vi "Get Output Uncertainty.vi"(8 "error in (no error)":errorcluster, 9 "Specified Uncertainty (0: 90-days)":u32(ring) items=["90-days", "365-days"], 10 "Output (T: Primary)":bool=TRUE, 11 "VISA resource name":refnum<visa-resource-name>) -> (0 "error out":errorcluster, 1 "Output Uncertainty Units":i32, 2 "Output Uncertainty":dbl format="%.4f", 3 "VISA resource name out":refnum<visa-resource-name>, 4 "Specification Interval":i32)   [LabVIEW 2013, in "Fluke 5XXX Series Multicalibrators.lvlib"]
doc: "This VI returns specified uncertainties for the present output. If there are no specifications for an output, returns value less or equal to zero."
uses:
  Fluke 5XXX Series Multicalibrators.lvlib
panel:
  # "Primary"
  # "Secondary"
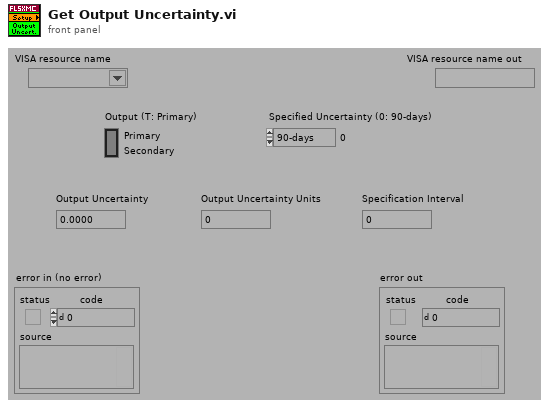
[diagram p1: front panel]
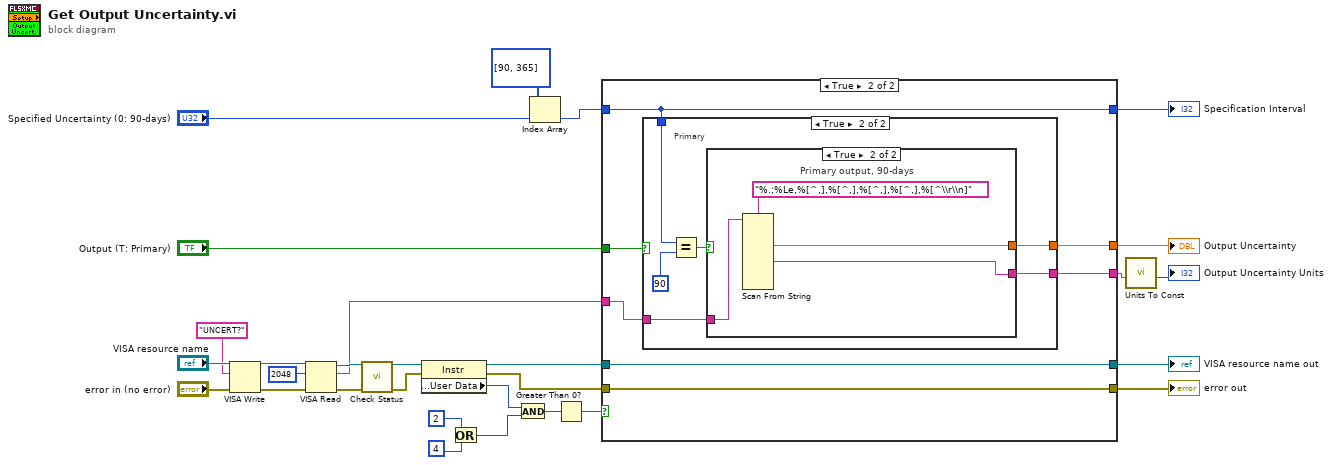
[diagram p0: block diagram]
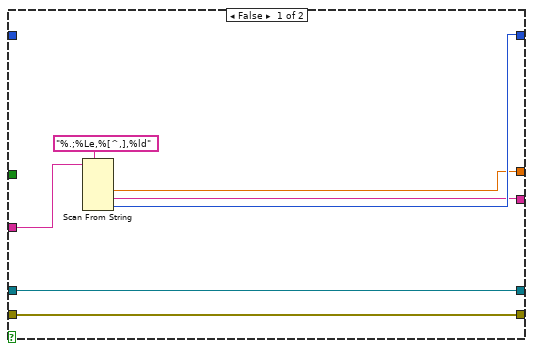
[diagram p2: hidden frame]
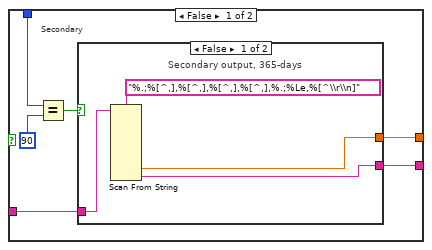
[diagram p3: hidden frame]
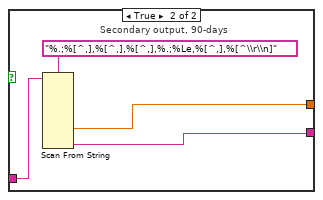
[diagram p4: hidden frame]
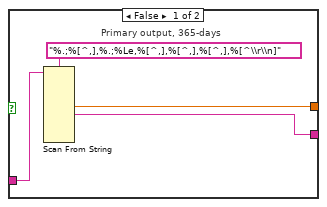
[diagram p5: hidden frame]
diagram:
  n1 = VISA Write(VISA resource name="VISA resource name", write buffer="UNCERT?", error in (no error)="error in (no error)") -> (VISA resource name out=w17:refnum<visa-resource-name>, error out=w16:errorcluster)  [unwired: 1 out]
  n2 = VISA Read(VISA resource name=w17, byte count=u32 2048 ("byte count (0)"), error in (no error)=w16) -> (VISA resource name out=w13:refnum<visa-resource-name>, read buffer=w10:string, error out=w14:errorcluster)  [unwired: 1 out]
  n3 = call "Check Status.vi"("VISA resource name"=w13, "error in (no error)"=w14) -> ("VISA resource name out"=w8:refnum<visa-resource-name>, "error out"=w6:errorcluster)  [unwired: 12 in]
  n4 = property class="Instr"(reference=w8, error in=w6) -> (reference out=w7:refnum<visa-resource-name>, error out=w5:errorcluster, "General Settings:User Data"=w4:u32)
  n5 = Or(x=u32 2 ("Numeric"), y=u32 4 ("Numeric")) -> (x .or. y?=w3:u32)
  n6 = And(x=w4, y=w3) -> (x .and. y?=w2:u32)
  n7 = Index Array(array=i32[] [90, 365] ("Specified Uncertainty arr"), index="Specified Uncertainty (0: 90-days)") -> (element=w27:i32)
  n8 = Greater Than 0?(x=w2) -> (x > 0?=w1:bool)
  n9 = case shown="True" w1 {
    tunnel: w27 -> [_ w41]
    tunnel: [w34 w41] -> w26
    tunnel: "Output (T: Primary)" -> [_ w43]
    tunnel: w10 -> [w35 w42]
    tunnel: w7 -> [w31 w37]
    tunnel: [w32 w40] -> w24
    tunnel: [w33 w39] -> w9
    tunnel: [w31 w37] -> w21
    tunnel: w5 -> [w30 w38]
    tunnel: [w30 w38] -> w22
    frame False {
      n10 = Scan From String(format string="%.;%Le,%[^,],%ld", input string=w35) -> (output 1=w32:dbl, output 2=w33:string, output 3=w34:i32)  [unwired: 5 in, 3 out]
    }
    frame True {
      n11 = case shown="True" w43 {
        tunnel: w42 -> [w47 w63]
        tunnel: w41 -> [w46 w60]
        tunnel: [w45 w59] -> w40
        tunnel: [w44 w58] -> w39
        frame False {
          # "Secondary"
          n12 = Equal?(x=w46, y=90) -> (x = y?=w49:bool)
          n13 = case shown="False" w49 {
            tunnel: w47 -> [w52 w56]
            tunnel: [w51 w55] -> w45
            tunnel: [w50 w54] -> w44
            frame False {
              # "Secondary output, 365-days"
              n14 = Scan From String(format string="%.;%[^,],%[^,],%[^,],%[^,],%.;%Le,%[^\\r\\n]", input string=w52) -> (output 5=w51:dbl, output 6=w50:string)  [unwired: 12 in, 3 out]
            }
            frame True {
              # "Secondary output, 90-days"
              n15 = Scan From String(format string="%.;%[^,],%[^,],%[^,],%.;%Le,%[^,],%[^\\r\\n]", input string=w56) -> (output 4=w55:dbl, output 6=w54:string)  [unwired: 12 in, 3 out]
            }
          }
        }
        frame True {
          # "Primary"
          n16 = Equal?(x=w60, y=90) -> (x = y?=w62:bool)
          n17 = case shown="True" w62 {
            tunnel: w63 -> [w66 w70]
            tunnel: [w65 w69] -> w59
            tunnel: [w64 w68] -> w58
            frame False {
              # "Primary output, 365-days"
              n18 = Scan From String(format string="%.;%[^,],%.;%Le,%[^,],%[^,],%[^,],%[^\\r\\n]", input string=w66) -> (output 2=w65:dbl, output 3=w64:string)  [unwired: 12 in, 3 out]
            }
            frame True {
              # "Primary output, 90-days"
              n19 = Scan From String(format string="%.;%Le,%[^,],%[^,],%[^,],%[^,],%[^\\r\\n]", input string=w70) -> (output 1=w69:dbl, output 3=w68:string)  [unwired: 12 in, 3 out]
            }
          }
        }
      }
    }
  }
  "Output Uncertainty" <- w24
  "Specification Interval" <- w26
  "VISA resource name out" <- w21
  "error out" <- w22
  n20 = call "Units To Const.vi"("Units"=w9) -> ("Const"=→"Output Uncertainty Units":i32)  [unwired: 10 in]
